vi "disable.vi"(8 "error in (no error)":errorcluster, 10 "model in":refnum<class "IModel.lvclass">, 11 "EnabledState in":refnum<class "EnabledState.lvclass">) -> (0 "error out":errorcluster, 2 "model out":refnum<class "IModel.lvclass">, 3 "EnabledState out":refnum<class "EnabledState.lvclass">)   [LabVIEW 2016, in "States.lvlib" / "EnabledState.lvclass"]
uses:
  EnabledState.lvclass
  IModel/IModel.lvclass
  Typedefs/CommandValue.ctl
  ts_sallv_sedspectrometer/DataTypes/logevent_summaryState.ctl
  ts_sallv_sedspectrometer/DataTypes/logevent_detailedState.ctl
  Typedefs/SEDSpectrometerTypedefs.lvlib
  ts_sallv_sedspectrometer/SALLV_sedSpectrometer.lvlib
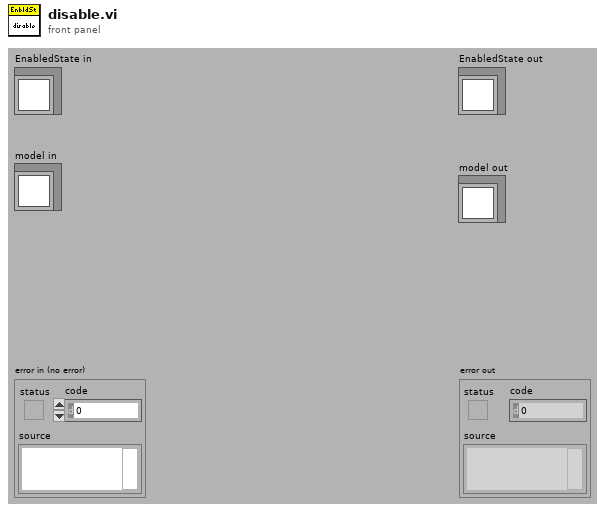
[diagram p1: front panel]
types:
  T1 = typedef "SALLV_sedSpectrometer.lvlib/logevent_detailedState.ctl" = cluster{"detailedState":enum32{"", "DisabledState", "EnabledState", "FaultState", "OfflineState", "StandbyState", "ImagingState", "NotImagingState"}, "priority":i32}
  T2 = typedef "SALLV_sedSpectrometer.lvlib/logevent_summaryState.ctl" = cluster{"summaryState":enum32{"", "DisabledState", "EnabledState", "FaultState", "OfflineState", "StandbyState"}, "priority":i32}
  T3 = typedef "SEDSpectrometerTypedefs.lvlib/CommandValue.ctl" = enum16{"clearError", "disable", "enable", "exit", "GoToStandby", "OnHeartbeat", "OnIncomingMessagingError", "OnInterrupt", "start", "captureSpectImage", "setSpectTempSetpoint", "stopImageCapture"}
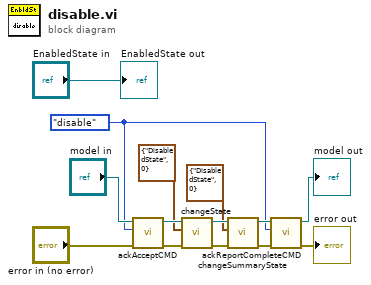
[diagram p0: block diagram]
diagram:
  w3 = CommandValue."disable" ("CommandValue")
  n1 = call-dynamic "ackAcceptCMD.vi"("error in (no error)"="error in (no error)", "CommandValue"=w3, "IModel in"="model in") -> ("error out"=w7:errorcluster, "IModel out"=w4:refnum<class "IModel.lvclass">)  [unwired: 7 in]
  n2 = call-dynamic "changeState.vi"("error in (no error)"=w7, "DetailedState"=T1 {"detailedState"=enum."DisabledState", "priority"=0} ("logevent_DetailedState"), "IModel in"=w4) -> ("error out"=w12:errorcluster, "IModel out"=w13:refnum<class "IModel.lvclass">)  [unwired: 7 in]
  n3 = call-dynamic "changeSummaryState.vi"("error in (no error)"=w12, "logevent_SummaryState"=T2 {"summaryState"=enum."DisabledState", "priority"=0}, "IModel in"=w13) -> ("error out"=w10:errorcluster, "IModel out"=w9:refnum<class "IModel.lvclass">)  [unwired: 7 in]
  n4 = call-dynamic "ackReportCompleteCMD.vi"("error in (no error)"=w10, "CommandValue"=w3, "IModel in"=w9) -> ("error out"=→"error out":errorcluster, "IModel out"=→"model out":refnum<class "IModel.lvclass">)  [unwired: 7 in]
  "EnabledState out" <- "EnabledState in"
